vi "Configuration Convert 1.1 to 1.2.vi"(8 "error in (no error)":errorcluster, 11 "framework configuration 1.1":T2={"Plugins"=[{"name"="Plugin", "components"=[], "cycle timing"={"priority"=10000, "decimation"=1, "offset"=0}, "threads"=[], "Transfer Groups"=[{"name"="Group", "direction"=enum."Tx", "cycle timing"={"priority"=100, "decimation"=1, "offset"=0}, "thread index"=-1, "settings"=[], "Transfers"=[{"name"="Transfer", "byte order"=enum."big-endian", "settings"=[], "channels"=[{"string offset"=0, "string data type"=enum."DBL", "engine data type"=enum."DBL", "name"="Channel", "settings"=[], "units"="V"}]}], "timeout behavior"=enum."Increment Late Count"}], "settings"=[]}]}) -> (0 "error out":errorcluster, 3 "framework configuration 1.2":T1={"plugins"=[{"name"="", "components"=[], "cycle timing"={"priority"=100, "decimation"=1, "offset"=0}, "threads"=[{"processor"=-2, "priority offset"=0, "settings"=[]}, {"processor"=-2, "priority offset"=0, "settings"=[]}, {"processor"=-2, "priority offset"=0, "settings"=[]}, {"processor"=-2, "priority offset"=0, "settings"=[]}], "transfer groups"=[{"name"="", "direction"=enum."Tx", "cycle timing"={"priority"=100, "decimation"=1, "offset"=0}, "thread index"=0, "settings"=[], "transfers"=[{"name"="", "byte order"=enum."big-endian", "settings"=[], "channels"=[]}], "timeout behavior"=enum."Increment Late Count"}], "settings"=[]}]})   [LabVIEW 2017, in "DSF Core.lvlib" / "Configuration Session.lvclass"]
uses:
  Configuration Session.lvclass
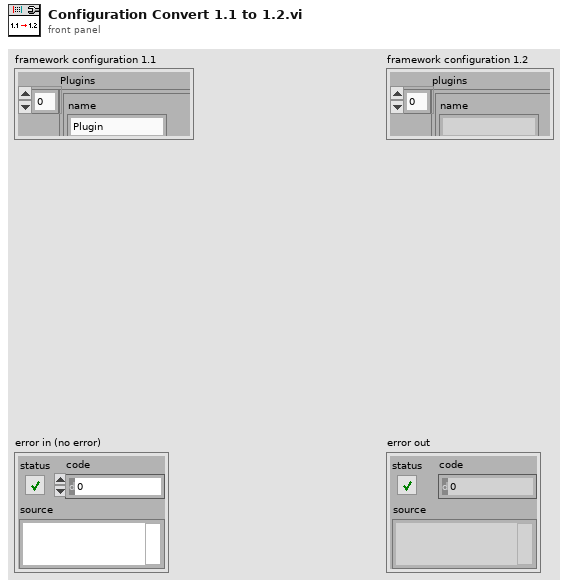
[diagram p1: front panel]
types:
  T1 = cluster{"plugins":cluster{"name":string, "components":string[], "cycle timing":cluster{"priority":u64, "decimation":u64, "offset":u64}, "threads":cluster{"processor":i32, "priority offset":i16, "settings":cluster{"component":string, "name":string, "values":cluster{"key":string, "value":string}[]}[]}[], "transfer groups":cluster{"name":string, "direction":enum8{"Tx", "Rx"}, "cycle timing":cluster{"priority":u64, "decimation":u64, "offset":u64}, "thread index":i32, "settings":cluster{"component":string, "name":string, "values":cluster{"key":string, "value":string}[]}[], "transfers":cluster{"name":string, "byte order":enum8{"big-endian", "little-endian"}, "settings":cluster{"component":string, "name":string, "values":cluster{"key":string, "value":string}[]}[], "channels":cluster{"string offset":u64, "name":string, "units":string, "engine data type":enum8{"Bool", "SGL", "DBL", "I8", "I16", "I32", "I64", "U8", "U16", "U32", "U64"}, "string data type":enum8{"Bool", "SGL", "DBL", "I8", "I16", "I32", "I64", "U8", "U16", "U32", "U64"}, "settings":cluster{"component":string, "name":string, "values":cluster{"key":string, "value":string}[]}[]}[]}[], "timeout behavior":enum8{"Increment Late Count", "Throw Error"}}[], "settings":cluster{"component":string, "name":string, "values":cluster{"key":string, "value":string}[]}[]}[]}
  T2 = cluster{"Plugins":cluster{"name":string, "components":string[], "cycle timing":cluster{"priority":u64, "decimation":u64, "offset":u64}, "threads":cluster{"buffer converter settings":cluster{"key":string, "value":string}[], "transceiver settings":cluster{"key":string, "value":string}[], "custom settings":cluster{"key":string, "value":string}[], "processor":i32, "priority offset":i16}[], "Transfer Groups":cluster{"name":string, "direction":enum8{"Tx", "Rx"}, "cycle timing":cluster{"priority":u64, "decimation":u64, "offset":u64}, "thread index":i32, "settings":cluster{"key":string, "value":string}[], "Transfers":cluster{"name":string, "byte order":enum8{"big-endian", "little-endian"}, "settings":cluster{"key":string, "value":string}[], "channels":cluster{"string offset":u64, "string data type":enum8{"Bool", "SGL", "DBL", "I8", "I16", "I32", "I64", "U8", "U16", "U32", "U64"}, "engine data type":enum8{"Bool", "SGL", "DBL", "I8", "I16", "I32", "I64", "U8", "U16", "U32", "U64"}, "name":string, "settings":cluster{"key":string, "value":string}[], "units":string}[]}[], "timeout behavior":enum8{"Increment Late Count", "Throw Error"}}[], "settings":cluster{"key":string, "value":string}[]}[]}
  T3 = cluster{"component":string, "name":string, "values":cluster{"key":string, "value":string}[]}
  T4 = cluster{"name":string, "components":string[], "cycle timing":cluster{"priority":u64, "decimation":u64, "offset":u64}, "threads":cluster{"processor":i32, "priority offset":i16, "settings":cluster{"component":string, "name":string, "values":cluster{"key":string, "value":string}[]}[]}[], "transfer groups":cluster{"name":string, "direction":enum8{"Tx", "Rx"}, "cycle timing":cluster{"priority":u64, "decimation":u64, "offset":u64}, "thread index":i32, "settings":cluster{"component":string, "name":string, "values":cluster{"key":string, "value":string}[]}[], "transfers":cluster{"name":string, "byte order":enum8{"big-endian", "little-endian"}, "settings":cluster{"component":string, "name":string, "values":cluster{"key":string, "value":string}[]}[], "channels":cluster{"string offset":u64, "name":string, "units":string, "engine data type":enum8{"Bool", "SGL", "DBL", "I8", "I16", "I32", "I64", "U8", "U16", "U32", "U64"}, "string data type":enum8{"Bool", "SGL", "DBL", "I8", "I16", "I32", "I64", "U8", "U16", "U32", "U64"}, "settings":cluster{"component":string, "name":string, "values":cluster{"key":string, "value":string}[]}[]}[]}[], "timeout behavior":enum8{"Increment Late Count", "Throw Error"}}[], "settings":cluster{"component":string, "name":string, "values":cluster{"key":string, "value":string}[]}[]}
  T5 = cluster{"name":string, "direction":enum8{"Tx", "Rx"}, "cycle timing":cluster{"priority":u64, "decimation":u64, "offset":u64}, "thread index":i32, "settings":cluster{"component":string, "name":string, "values":cluster{"key":string, "value":string}[]}[], "transfers":cluster{"name":string, "byte order":enum8{"big-endian", "little-endian"}, "settings":cluster{"component":string, "name":string, "values":cluster{"key":string, "value":string}[]}[], "channels":cluster{"string offset":u64, "name":string, "units":string, "engine data type":enum8{"Bool", "SGL", "DBL", "I8", "I16", "I32", "I64", "U8", "U16", "U32", "U64"}, "string data type":enum8{"Bool", "SGL", "DBL", "I8", "I16", "I32", "I64", "U8", "U16", "U32", "U64"}, "settings":cluster{"component":string, "name":string, "values":cluster{"key":string, "value":string}[]}[]}[]}[], "timeout behavior":enum8{"Increment Late Count", "Throw Error"}}
  T6 = cluster{"name":string, "byte order":enum8{"big-endian", "little-endian"}, "settings":cluster{"component":string, "name":string, "values":cluster{"key":string, "value":string}[]}[], "channels":cluster{"string offset":u64, "name":string, "units":string, "engine data type":enum8{"Bool", "SGL", "DBL", "I8", "I16", "I32", "I64", "U8", "U16", "U32", "U64"}, "string data type":enum8{"Bool", "SGL", "DBL", "I8", "I16", "I32", "I64", "U8", "U16", "U32", "U64"}, "settings":cluster{"component":string, "name":string, "values":cluster{"key":string, "value":string}[]}[]}[]}
  T7 = cluster{"string offset":u64, "name":string, "units":string, "engine data type":enum8{"Bool", "SGL", "DBL", "I8", "I16", "I32", "I64", "U8", "U16", "U32", "U64"}, "string data type":enum8{"Bool", "SGL", "DBL", "I8", "I16", "I32", "I64", "U8", "U16", "U32", "U64"}, "settings":cluster{"component":string, "name":string, "values":cluster{"key":string, "value":string}[]}[]}
  T8 = cluster{"processor":i32, "priority offset":i16, "settings":cluster{"component":string, "name":string, "values":cluster{"key":string, "value":string}[]}[]}
  T9 = cluster{"name":string, "components":string[], "cycle timing":cluster{"priority":u64, "decimation":u64, "offset":u64}, "threads":cluster{"buffer converter settings":cluster{"key":string, "value":string}[], "transceiver settings":cluster{"key":string, "value":string}[], "custom settings":cluster{"key":string, "value":string}[], "processor":i32, "priority offset":i16}[], "Transfer Groups":cluster{"name":string, "direction":enum8{"Tx", "Rx"}, "cycle timing":cluster{"priority":u64, "decimation":u64, "offset":u64}, "thread index":i32, "settings":cluster{"key":string, "value":string}[], "Transfers":cluster{"name":string, "byte order":enum8{"big-endian", "little-endian"}, "settings":cluster{"key":string, "value":string}[], "channels":cluster{"string offset":u64, "string data type":enum8{"Bool", "SGL", "DBL", "I8", "I16", "I32", "I64", "U8", "U16", "U32", "U64"}, "engine data type":enum8{"Bool", "SGL", "DBL", "I8", "I16", "I32", "I64", "U8", "U16", "U32", "U64"}, "name":string, "settings":cluster{"key":string, "value":string}[], "units":string}[]}[], "timeout behavior":enum8{"Increment Late Count", "Throw Error"}}[], "settings":cluster{"key":string, "value":string}[]}[]
  T10 = cluster{"priority":u64, "decimation":u64, "offset":u64}
  T11 = cluster{"buffer converter settings":cluster{"key":string, "value":string}[], "transceiver settings":cluster{"key":string, "value":string}[], "custom settings":cluster{"key":string, "value":string}[], "processor":i32, "priority offset":i16}[]
  T12 = cluster{"name":string, "direction":enum8{"Tx", "Rx"}, "cycle timing":cluster{"priority":u64, "decimation":u64, "offset":u64}, "thread index":i32, "settings":cluster{"key":string, "value":string}[], "Transfers":cluster{"name":string, "byte order":enum8{"big-endian", "little-endian"}, "settings":cluster{"key":string, "value":string}[], "channels":cluster{"string offset":u64, "string data type":enum8{"Bool", "SGL", "DBL", "I8", "I16", "I32", "I64", "U8", "U16", "U32", "U64"}, "engine data type":enum8{"Bool", "SGL", "DBL", "I8", "I16", "I32", "I64", "U8", "U16", "U32", "U64"}, "name":string, "settings":cluster{"key":string, "value":string}[], "units":string}[]}[], "timeout behavior":enum8{"Increment Late Count", "Throw Error"}}[]
  T13 = cluster{"component":string, "name":string, "values":cluster{"key":string, "value":string}[]}[]
  T14 = cluster{"name":string, "byte order":enum8{"big-endian", "little-endian"}, "settings":cluster{"key":string, "value":string}[], "channels":cluster{"string offset":u64, "string data type":enum8{"Bool", "SGL", "DBL", "I8", "I16", "I32", "I64", "U8", "U16", "U32", "U64"}, "engine data type":enum8{"Bool", "SGL", "DBL", "I8", "I16", "I32", "I64", "U8", "U16", "U32", "U64"}, "name":string, "settings":cluster{"key":string, "value":string}[], "units":string}[]}[]
  T15 = cluster{"string offset":u64, "string data type":enum8{"Bool", "SGL", "DBL", "I8", "I16", "I32", "I64", "U8", "U16", "U32", "U64"}, "engine data type":enum8{"Bool", "SGL", "DBL", "I8", "I16", "I32", "I64", "U8", "U16", "U32", "U64"}, "name":string, "settings":cluster{"key":string, "value":string}[], "units":string}[]
  T16 = enum8{"Bool", "SGL", "DBL", "I8", "I16", "I32", "I64", "U8", "U16", "U32", "U64"}
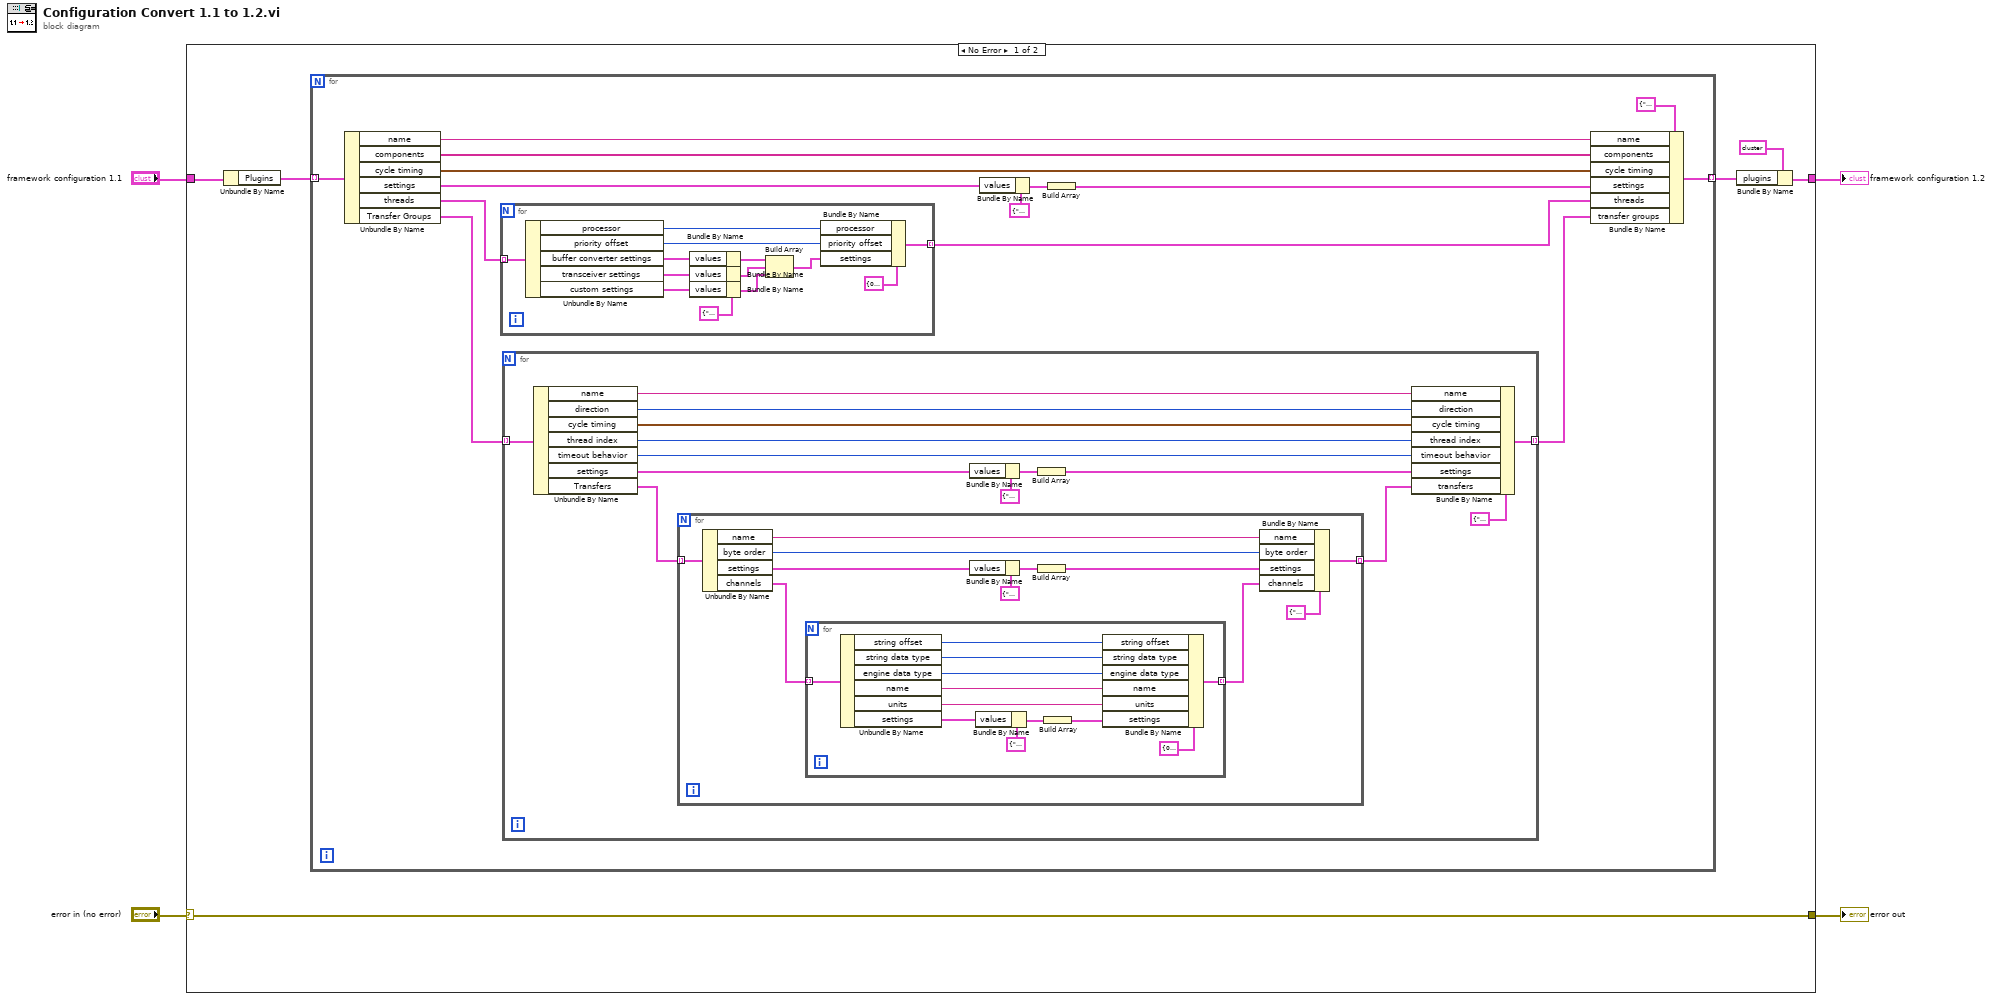
[diagram p0: block diagram]
diagram:
  n1 = case shown="No Error" "error in (no error)" {
    selector: "error in (no error)" -> [w10 w75]
    tunnel: [w10 w75] -> w4
    tunnel: "framework configuration 1.1" -> [w9 _]
    tunnel: [w6 _] -> w1
    frame No Error {
      n2 = Unbundle By Name(w9) -> ("Plugins"=w8:T9)
      n3 = for {
        tunnel: w8 -> [w24] mode=indexing
        tunnel: [w22] -> w5 mode=indexing
        n4 = Unbundle By Name(w24) -> ("name"=w21:string, "components"=w20:string[], "cycle timing"=w19:T10, "settings"=w12:cluster{"key":string, "value":string}[], "threads"=w15:T11, "Transfer Groups"=w17:T12)
        n5 = for {
          tunnel: w15 -> [w74] mode=indexing
          tunnel: [w62] -> w18 mode=indexing
          w64 = T3 {"component"="", "name"="", "values"=[]} ("settings")
          n6 = Unbundle By Name(w74) -> ("processor"=w72:i32, "priority offset"=w66:i16, "buffer converter settings"=w69:cluster{"key":string, "value":string}[], "transceiver settings"=w70:cluster{"key":string, "value":string}[], "custom settings"=w71:cluster{"key":string, "value":string}[])
          n7 = Bundle By Name(cluster=w64, "values"=w69) -> (w65:T3)
          n8 = Bundle By Name(cluster=w64, "values"=w70) -> (w68:T3)
          n9 = Bundle By Name(cluster=w64, "values"=w71) -> (w67:T3)
          n10 = Build Array(w65, w68, w67) -> (w63:T13)
          n11 = Bundle By Name(cluster=T8 {"processor"=0, "priority offset"=0, "settings"=[]} ("Plugin Thread Configuration"), "processor"=w72, "priority offset"=w66, "settings"=w63) -> (w62:T8)
        }
        n12 = for {
          tunnel: w17 -> [w38] mode=indexing
          tunnel: [w37] -> w16 mode=indexing
          n13 = Unbundle By Name(w38) -> ("name"=w35:string, "direction"=w34:enum8{"Tx", "Rx"}, "cycle timing"=w33:T10, "thread index"=w32:i32, "timeout behavior"=w31:enum8{"Increment Late Count", "Throw Error"}, "settings"=w26:cluster{"key":string, "value":string}[], "Transfers"=w30:T14)
          n14 = for {
            tunnel: w30 -> [w49] mode=indexing
            tunnel: [w45] -> w29 mode=indexing
            n15 = Unbundle By Name(w49) -> ("name"=w47:string, "byte order"=w46:enum8{"big-endian", "little-endian"}, "settings"=w43:cluster{"key":string, "value":string}[], "channels"=w40:T15)
            n16 = for {
              tunnel: w40 -> [w60] mode=indexing
              tunnel: [w50] -> w39 mode=indexing
              n17 = Unbundle By Name(w60) -> ("string offset"=w59:u64, "string data type"=w58:T16, "engine data type"=w57:T16, "name"=w56:string, "units"=w55:string, "settings"=w52:cluster{"key":string, "value":string}[])
              n18 = Bundle By Name(cluster=T3 {"component"="", "name"="", "values"=[]} ("settings"), "values"=w52) -> (w53:T3)
              n19 = Build Array(w53) -> (w51:T13)
              n20 = Bundle By Name(cluster=T7 {"string offset"=0, "name"="", "units"="", "engine data type"=enum."Bool", "string data type"=enum."Bool", "settings"=[]} ("channel configuration"), "string offset"=w59, "string data type"=w58, "engine data type"=w57, "name"=w56, "units"=w55, "settings"=w51) -> (w50:T7)
            }
            n21 = Bundle By Name(cluster=T3 {"component"="", "name"="", "values"=[]} ("settings"), "values"=w43) -> (w44:T3)
            n22 = Build Array(w44) -> (w41:T13)
            n23 = Bundle By Name(cluster=T6 {"name"="", "byte order"=enum."big-endian", "settings"=[], "channels"=[]} ("Transfer Configuration"), "name"=w47, "byte order"=w46, "settings"=w41, "channels"=w39) -> (w45:T6)
          }
          n24 = Bundle By Name(cluster=T3 {"component"="", "name"="", "values"=[]} ("settings"), "values"=w26) -> (w27:T3)
          n25 = Build Array(w27) -> (w25:T13)
          n26 = Bundle By Name(cluster=T5 {"name"="", "direction"=enum."Tx", "cycle timing"={"priority"=0, "decimation"=0, "offset"=0}, "thread index"=0, "settings"=[], "transfers"=[], "timeout behavior"=enum."Increment Late Count"} ("Transfer Group Configuration"), "name"=w35, "direction"=w34, "cycle timing"=w33, "thread index"=w32, "timeout behavior"=w31, "settings"=w25, "transfers"=w29) -> (w37:T5)
        }
        n27 = Bundle By Name(cluster=T3 {"component"="", "name"="", "values"=[]} ("settings"), "values"=w12) -> (w13:T3)
        n28 = Build Array(w13) -> (w11:T13)
        n29 = Bundle By Name(cluster=T4 {"name"="", "components"=[], "cycle timing"={"priority"=0, "decimation"=0, "offset"=0}, "threads"=[], "transfer groups"=[], "settings"=[]} ("Plugin Configuration"), "name"=w21, "components"=w20, "cycle timing"=w19, "settings"=w11, "threads"=w18, "transfer groups"=w16) -> (w22:T4)
      }
      n30 = Bundle By Name(cluster=T1 {"plugins"=[{"name"="", "components"=[], "cycle timing"={"priority"=100, "decimation"=1, "offset"=0}, "threads"=[{"processor"=-2, "priority offset"=0, "settings"=[]}, {"processor"=-2, "priority offset"=0, "settings"=[]}, {"processor"=-2, "priority offset"=0, "settings"=[]}, {"processor"=-2, "priority offset"=0, "settings"=[]}], "transfer groups"=[{"name"="", "direction"=enum."Tx", "cycle timing"={"priority"=100, "decimation"=1, "offset"=0}, "thread index"=0, "settings"=[], "transfers"=[{"name"="", "byte order"=enum."big-endian", "settings"=[], "channels"=[]}], "timeout behavior"=enum."Increment Late Count"}], "settings"=[]}]} ("framework configuration 1.2"), "plugins"=w5) -> (w6:T1)
    }
    frame Error {
    }
  }
  "error out" <- w4
  "framework configuration 1.2" <- w1
